vi "Get DIO Bits To Inhibit Motion Status.vi"(4 "error in (no error)":errorcluster, 6 "Axis (1)":i32=1 min=1 max=3, 7 "VISA resource name":refnum<visa-resource-name>) -> (0 "error out":errorcluster, 2 "DIO Bits  Motion Status Inhibition":bool, 3 "VISA resource name out":refnum<visa-resource-name>)   [LabVIEW 2018, in "Newport ESP301.lvlib"]
doc: "Reads the status (enable/disable) of inhibit motion through DIO bits.\n\n<B>DIO Bits Motion Status Inhibition</B> : T:enable, F:disable"
uses:
  Newport ESP301.lvlib
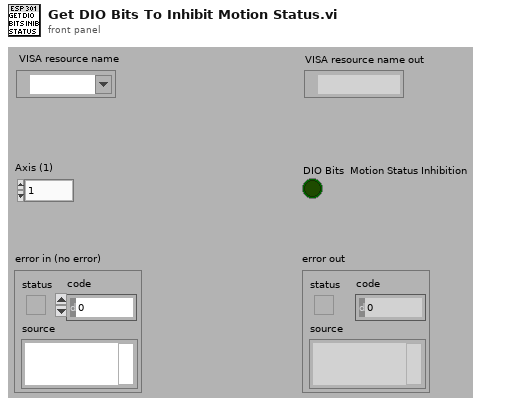
[diagram p1: front panel]
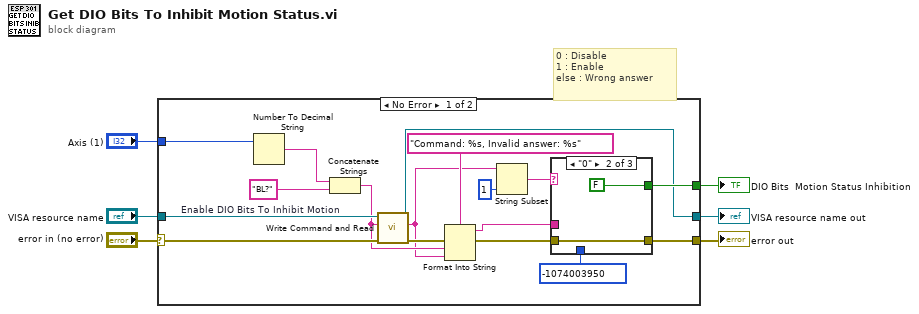
[diagram p0: block diagram]
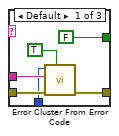
[diagram p2: hidden frame]
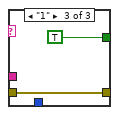
[diagram p3: hidden frame]
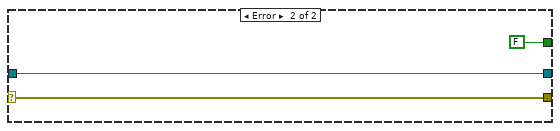
[diagram p4: hidden frame]
diagram:
  # "0 : Disable\n1 : Enable\nelse : Wrong answer"
  n1 = case shown="No Error" "error in (no error)" {
    selector: "error in (no error)" -> [w22 w36]
    tunnel: [w16 w36] -> w6
    tunnel: "VISA resource name" -> [w23 w35]
    tunnel: [w8 w35] -> w5
    tunnel: "Axis (1)" -> [w19 _]
    tunnel: [w15 FALSE ("Motion Done")] -> w1
    frame No Error {
      w20 = "BL?"  # Enable DIO Bits To Inhibit Motion
      n2 = Number To Decimal String(number=w19) -> (decimal integer string=w21:string)  [unwired: 1 out]
      n3 = Concatenate Strings(w21, w20) -> (w12:string)
      n4 = call "Write Command and Read.vi"("error in (no error)"=w22, "Command"=w12, "VISA resource name"=w23) -> ("error out"=w18:errorcluster, "Returned string"=w11:string, "VISA resource name out"=w8:refnum<visa-resource-name>)  [unwired: 2 in, 2 out]
      n5 = Format Into String(format string="Command: %s, Invalid answer: %s" ("error message (\"\")"), error in=w18, w12, w11) -> (resulting string=w10:string, error out=w17:errorcluster)  [unwired: 1 in]
      n6 = String Subset(string=w11, length (rest)=1 ("longueur (reste)")) -> (substring=w13:string)  [unwired: 1 out]
      n7 = case shown="\"0\"" w13 {
        tunnel: [w28 w30 w32] -> w16
        tunnel: [FALSE ("Motion Done") FALSE ("Motion Done") TRUE ("Motion Done")] -> w15
        tunnel: w17 -> [w26 w30 w32]
        tunnel: w10 -> [w25 _ _]
        tunnel: -1074003950 ("error code (0)") -> [w24 _ _]
        frame Default {
          n8 = call <vilib>:"Error Cluster From Error Code.vi"("show call chain? (False)"=TRUE, "error in (no error)"=w26, "error message (\"\")"=w25, "error code (0)"=w24) -> ("error out"=w28:errorcluster)  [unwired: 5 out]
        }
        frame "0" {
        }
        frame "1" {
        }
      }
    }
    frame Error {
    }
  }
  "error out" <- w6
  "VISA resource name out" <- w5
  "DIO Bits  Motion Status Inhibition" <- w1
